vi "Oxford-1820-Main-Launcher.vi"() -> ()   [LabVIEW 2019]
doc: "This VI will launch the PPMS 2 Instrument backend that will contunously monitor the state of the instrument and log to the DSC. The user has the option of launching a user interface (default) or allowing the backend to run headless. Run \"Launch PPMS2 UI.vi\" here or on a different computer to have a remote user interface. You can also use the APIs like \"Get Temperturature\" interact programmatically with the PPMS 2 Instrument backend."
uses:
  <vilib>/JKI/JKI SMO/SMO/Typedefs/SMOState --Enum.ctl
  SMOs/Instrument.Oxford1820/Instrument.Oxford1820.lvclass
  C:/Program Files (x86)/National Instruments/LabVIEW 2019/vi.lib/JKI/JKI SMO/SMO/SMO.lvclass
  C:/Program Files (x86)/National Instruments/LabVIEW 2019/user.lib/LevyLab/Instrument Framework/SMOs/Instrument/Instrument.lvclass
  SMOs/Instrument.Oxford1820 UI/Instrument UI.Oxford1820.lvclass
  C:/Program Files (x86)/National Instruments/LabVIEW 2019/vi.lib/JKI/JKI SMO/SMO.UI/SMO.UI.lvclass
  C:/Program Files (x86)/National Instruments/LabVIEW 2019/user.lib/LevyLab/Instrument Framework/SMOs/Instrument UI/Instrument UI.lvclass
  <vilib>/JKI/JKI SMO/SMO/SMO.lvclass/SMO.ctl
  <vilib>/JKI/JKI SMO/SMO.UI/SMO.UI.lvclass/SMO.UI.ctl
  <vilib>/JKI/JKI SMO/SMO/Private/ReftoDVR--SMO.vi
  <vilib>/JKI/JKI SMO/SMO.UI/SMO.UI.ReftoDVR.vi
  <vilib>/JKI/JKI SMO/SMO/SMO.lvclass
  <vilib>/JKI/JKI SMO/SMO.UI/SMO.UI.lvclass
  <userlib>/LevyLab/Instrument Framework/SMOs/Instrument UI/Instrument UI.lvclass
panel:
  in  "Debug Mode?":bool
  in  "Stop":bool=TRUE
  in  "Start":bool=TRUE
  in  "Splash Status":string="Push Start to Start..." caption="String"
  out "UI SMO State":T1=enum."Stopped"
  out "SMO State":T1
  out "error out":errorcluster
  # "OI 1820"
  # "v"
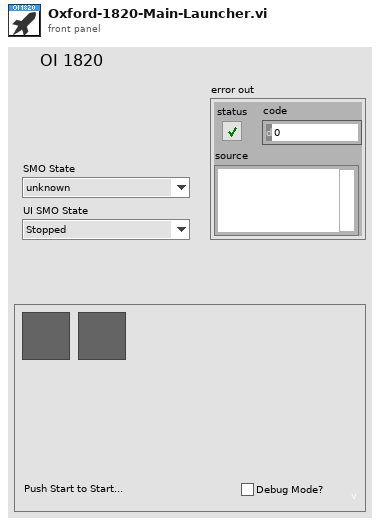
[diagram p1: front panel]
types:
  T1 = typedef "SMO.lvclass/SMOState --Enum.ctl" = enum16{"unknown", "Created", "Started", "Stopped"}
  T2 = enum32{"Invalid", "Standard", "Closed", "Hidden", "Minimized", "Maximized"}
  T3 = enum32{"invalid app kind", "Development System", "Run Time System", "Student Edition", "Embedded LabVIEW", "Evaluation", "Custom"}
  T4 = cluster{"Core":cluster{"Current VI Reference":refnum<vi>, "Close Panel on Exit?":bool}, "Instrument.Oxford1820":refnum<class "Instrument.Oxford1820.lvclass">, "Instrument.Oxford1820 UI":refnum<class "Instrument UI.Oxford1820.lvclass">}
  T5 = cluster{"Current VI Reference":refnum<vi>, "Close Panel on Exit?":bool}
  T6 = typedef "SMO.lvclass/Public Events.ctl" = cluster{"Error":refnum<user-event>, "State":refnum<user-event>, "Reserve State":refnum<user-event>}
  T7 = typedef "SMO.UI.lvclass/PublicEvents--Cluster.ctl" = cluster{"UI Hidden":refnum<user-event>, "UI State":refnum<user-event>}
  T8 = cluster{"Event Registration Refnum":refnum<event-registration>, "Event Registration Refnum":refnum<event-registration>}
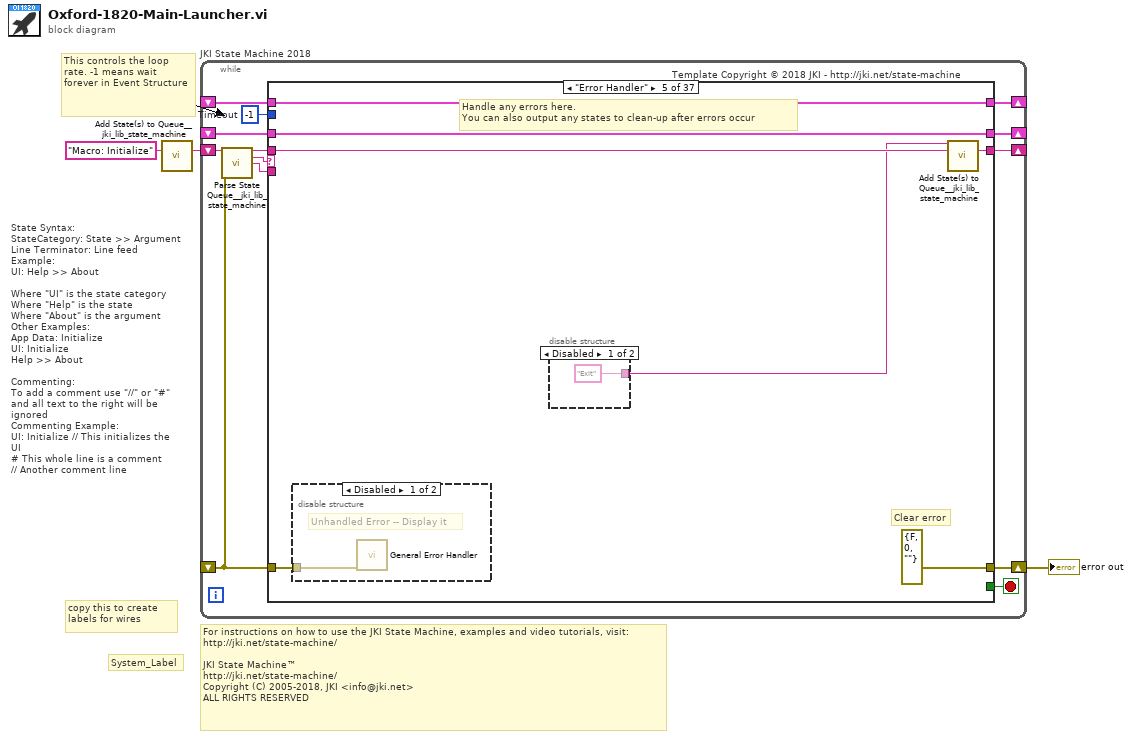
[diagram p0: block diagram]
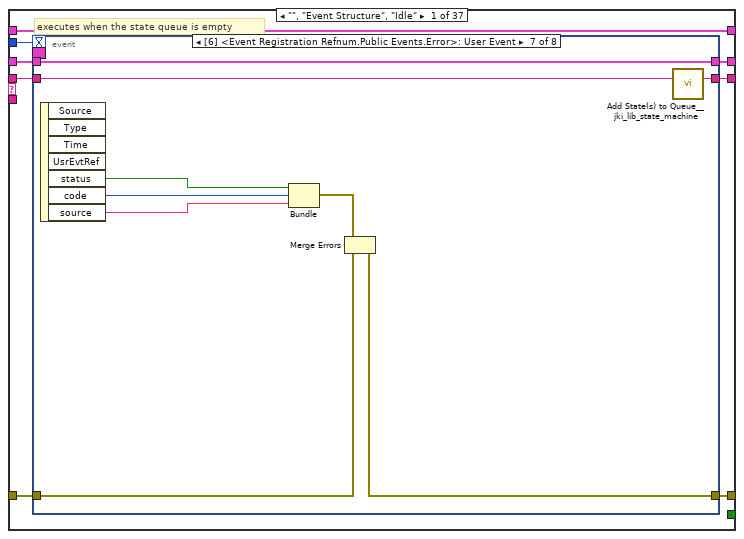
[diagram p2: hidden frame]
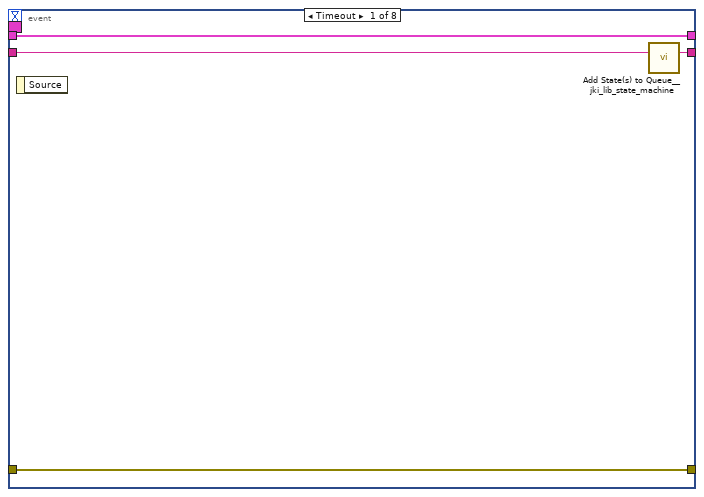
[diagram p3: hidden frame]
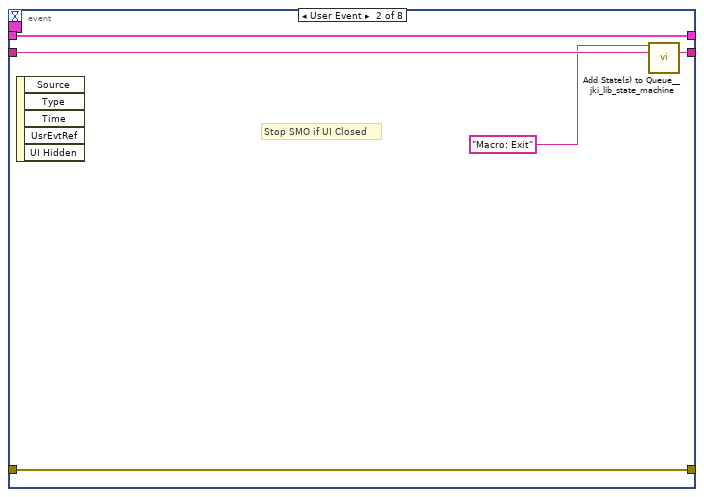
[diagram p4: hidden frame]
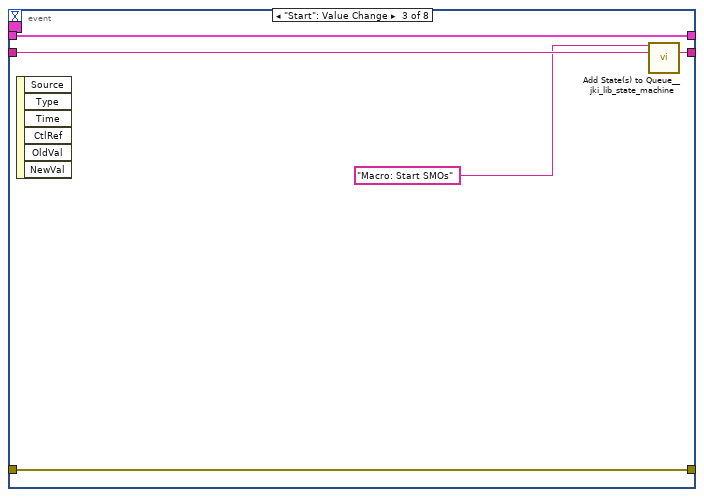
[diagram p5: hidden frame]
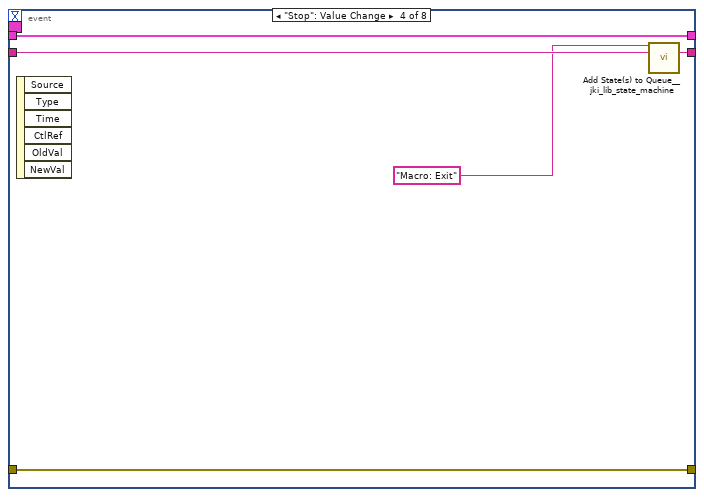
[diagram p6: hidden frame]
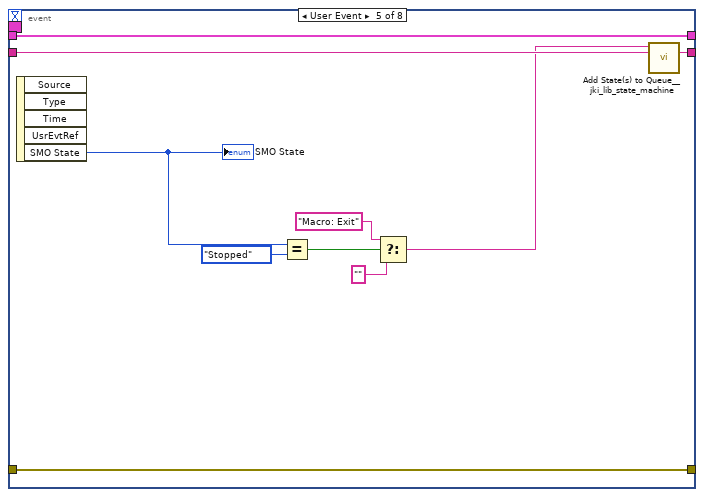
[diagram p7: hidden frame]
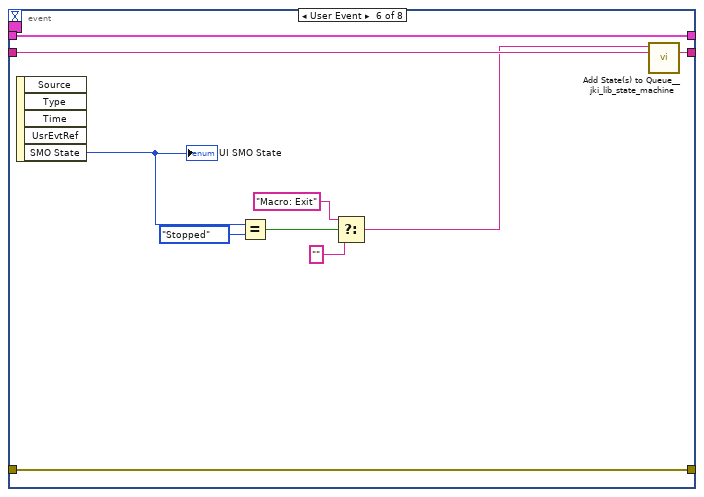
[diagram p8: hidden frame]
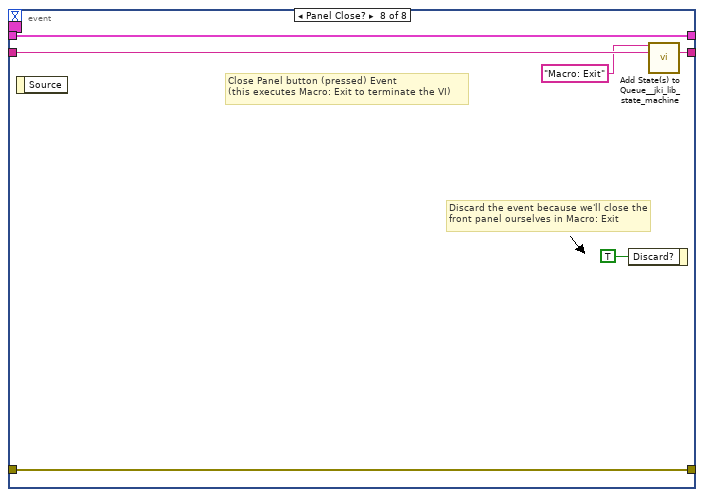
[diagram p9: hidden frame]
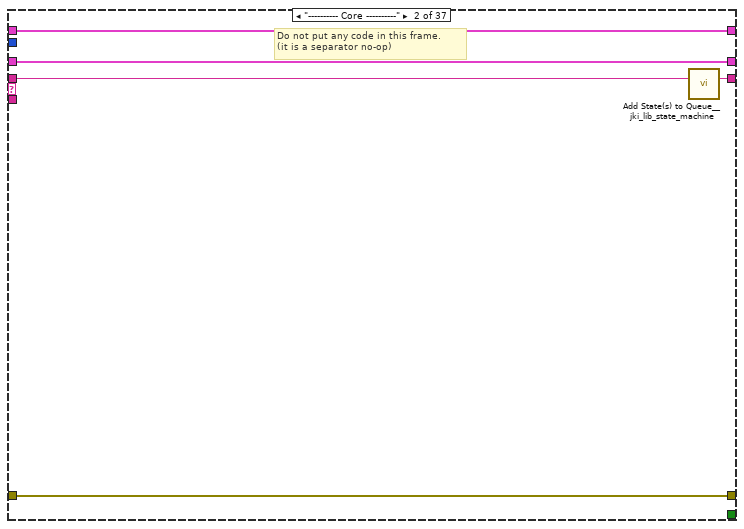
[diagram p10: hidden frame]
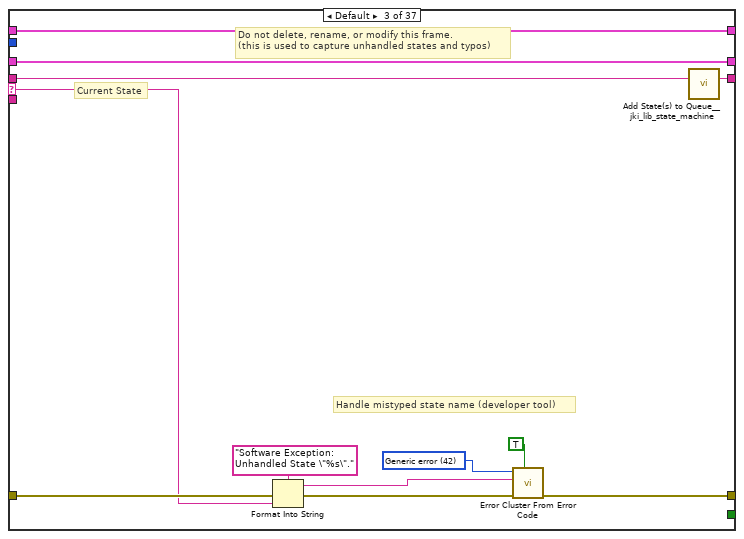
[diagram p11: hidden frame]
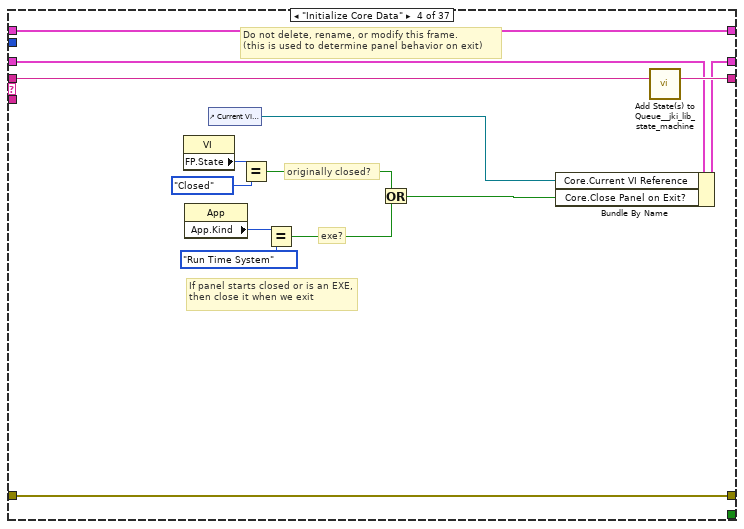
[diagram p12: hidden frame]
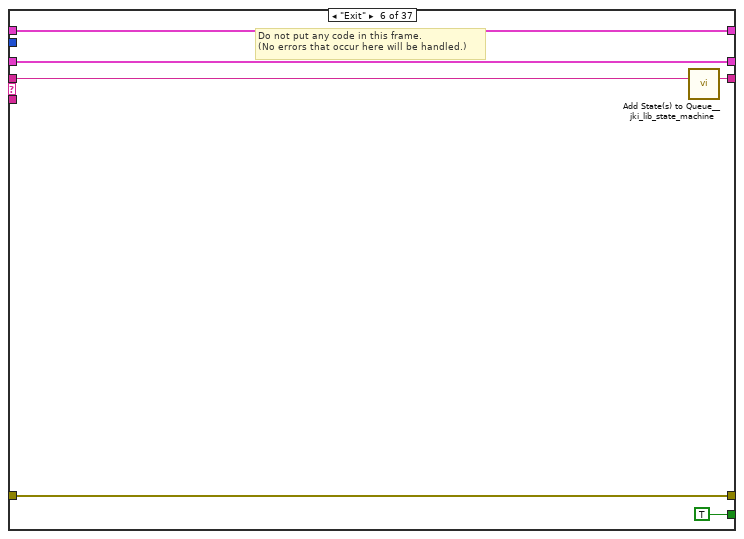
[diagram p15: hidden frame]
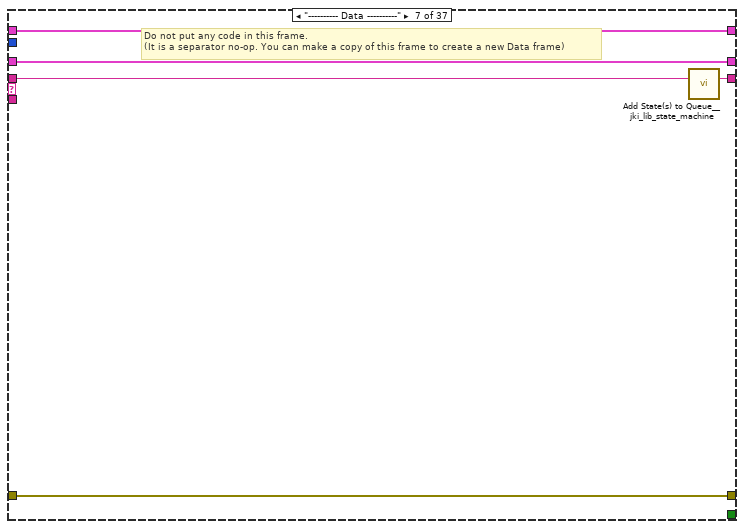
[diagram p16: hidden frame]
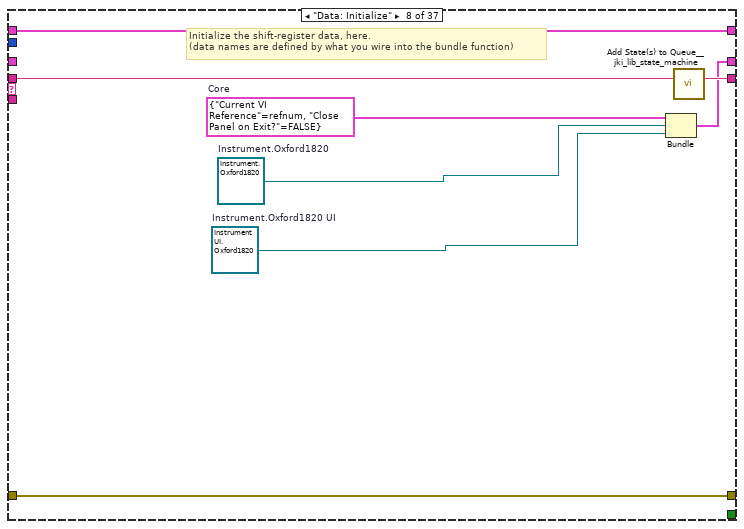
[diagram p17: hidden frame]
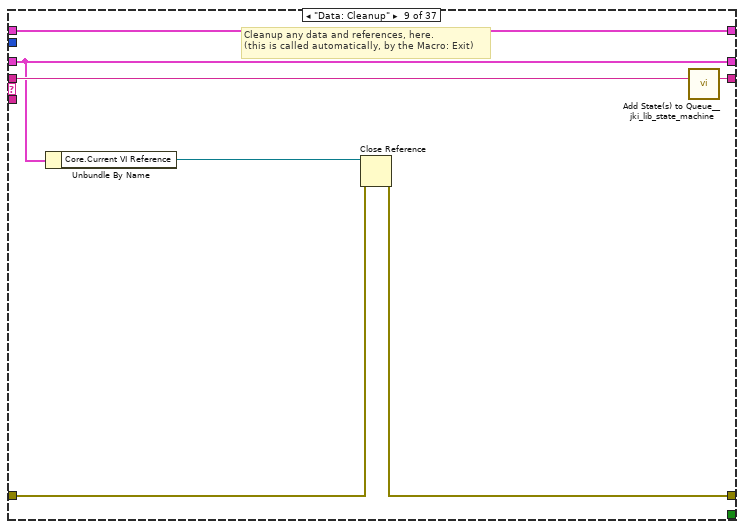
[diagram p18: hidden frame]
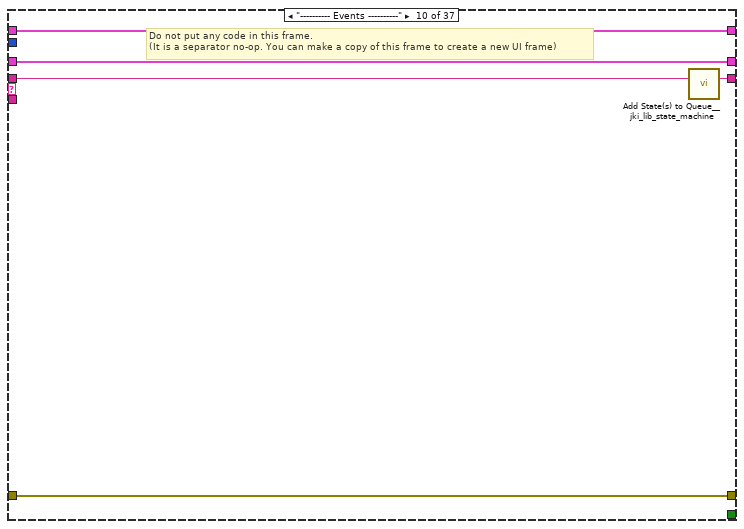
[diagram p19: hidden frame]
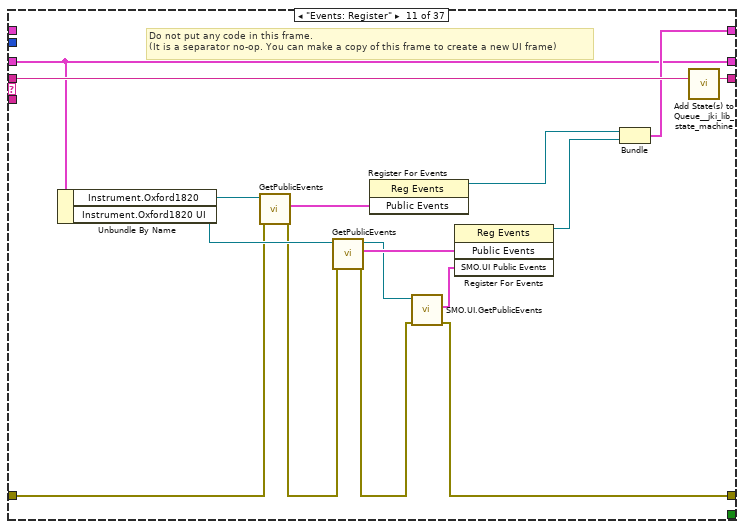
[diagram p20: hidden frame]
diagram:
  # "For instructions on how to use the JKI State Machine, examples and video tutorials, visit:\nhttp://jki.net/state-machine/\n\nJKI State Machine™\nhttp://jki.net/state-machine/\nCopyright (C) 2005-2018, JKI <info@jki.net>\nALL RIGHTS RESERVED"
  # "State Syntax:\nStateCategory: State >> Argument\nLine Terminator: Line feed\nExample:\nUI: Help >> About\n\nWhere \"UI\" is the state category\nWhere \"Help\" is the state\nWhere \"About\" is the argument\nOther Examples:\nApp Data: Initialize\nUI: Initialize\nHelp >> About\n\nCommenting:\nTo add a comment use \"//\" or \"#\" and all text to the right will be ignored\nCommenting Example:\nUI: Initialize // This initializes the UI\n# This whole line is a comment\n// Another comment line"
  # "copy this to create labels for wires"
  # "This controls the loop rate. -1 means wait forever in Event Structure"
  # "System_Label"
  n1 = call <vilib>:"Add State(s) to Queue__jki_lib_state_machine.vi"("State(s) in (\"\")"="Macro: Initialize") -> ("States Out"=w3:string)  [unwired: 14 in]
  n2 = while "JKI State Machine 2018" {
    shift-right: [w9] -> _
    shift-left: _ -> [w4]
    shift-right: [w12] -> w1
    shift-left: _ -> [w7]
    shift-right: [w11] -> _
    shift-left: w3 -> [w13]
    shift-right: [w6] -> _
    shift-left: _ -> [w5]
    stop <- w10 stop-if-true
    w8 = -1  # Timeout
    # "Template Copyright © 2018 JKI - http://jki.net/state-machine"
    n3 = call <vilib>:"Parse State Queue__jki_lib_state_machine.vi"("State Queue"=w13, "Error In (no error)"=w7) -> ("Remaining States"=w15:string, "Current State"=w16:string, "Arguments"=w14:string)  [unwired: 11 in]
    n4 = case shown="\"Error Handler\"" w16 {
      selector: w16 -> [_ _ w85 _ _ _ _ _ _ _ _ _ _ _ _ _ _ _ _ _ _ _ _ _ _ _ _ _ _ _ _ _ _ _ _ _ _]
      tunnel: w15 -> [w24 w83 w89 w109 w116 w124 w129 w137 w144 w149 w165 w171 w176 w182 w189 w201 w279 w284 w289 w295 w301 w307 w319 w324 w335 w344 w355 w370 w384 w391 w402 w417 w432 w447 w456 w463 w468]
      tunnel: w14 -> [_ _ _ _ _ _ _ _ _ _ _ _ _ _ w184 w195 _ _ _ _ _ _ _ _ _ _ _ _ _ _ _ _ _ _ _ w460 _]
      tunnel: [w21 w81 w91 w106 errorcluster {"status"=FALSE, "code"=0, "source"=""} ("error out") w121 w127 w134 w140 w147 w150 w166 w174 w177 w185 w198 w269 w282 w287 w293 w299 w305 w317 w322 w325 w337 w351 w366 w376 w385 w398 w413 w429 w444 w454 w458 w466] -> w12
      tunnel: w7 -> [w20 w81 w90 w106 w112 w121 w127 w134 w141 w147 w156 w167 w174 w179 w186 w199 w270 w282 w287 w293 w299 w305 w317 w322 w329 w338 w347 w362 w377 w386 w395 w410 w427 w440 w454 w459 w466]
      tunnel: [w23 w82 w88 w108 w115 w123 w128 w136 w143 w148 w164 w170 w175 w181 w188 w200 w278 w283 w288 w294 w300 w306 w318 w323 w334 w343 w354 w369 w383 w390 w401 w416 w431 w446 w455 w462 w467] -> w11
      tunnel: [_ _ _ _ _ TRUE _ _ _ _ _ _ _ _ _ _ _ _ _ _ _ _ _ _ _ _ _ _ _ _ _ _ _ _ _ _ _] -> w10
      tunnel: [w19 w80 w87 w107 w113 w122 w126 w135 w139 w146 w159 w169 w173 w180 w187 w197 w267 w281 w286 w292 w298 w304 w316 w321 w332 w339 w352 w367 w380 w388 w399 w414 w428 w443 w453 w461 w465] -> w9
      tunnel: w8 -> [w18 _ _ _ _ _ _ _ _ _ _ _ _ _ _ _ _ _ _ _ _ _ _ _ _ _ _ _ _ _ _ _ _ _ _ _ _]
      tunnel: [w17 w79 w84 w96 w110 w119 w125 w132 w138 w145 w162 w168 w172 w178 w183 w194 w268 w280 w285 w290 w297 w303 w310 w320 w333 w342 w353 w368 w382 w389 w400 w415 w430 w445 w452 w457 w464] -> w6
      tunnel: w5 -> [w17 w79 w84 w96 w110 w119 w125 w132 w138 w145 _ w168 w172 w178 w183 w194 w268 w280 w285 w290 w297 w303 w310 w320 w333 w342 w353 w368 w382 w389 w400 w415 w430 w445 w452 w457 w464]
      tunnel: w4 -> [w22 w80 w87 w102 w113 w122 w126 _ w139 w146 w159 w169 w173 w180 w187 w197 w267 w281 w286 w292 w298 w304 w316 w321 w331 w340 w352 w367 w381 w388 w399 w414 w428 w443 w453 w461 w465]
      frame "", "Event Structure", "Idle" {
        # "executes when the state queue is empty"
        n5 = event shown="[6] <Event Registration Refnum.Public Events.Error>: User Event" {
          selector: w17 -> [_ _ _ _ _ _ _ _]
          dyn-events: _ -> [_ _ _ _ _ _ _ _]
          timeout: w18 -> [_ _ _ _ _ _ _ _]
          tunnel: w24 -> [w28 w33 w38 w43 w53 w63 w72 w78]
          tunnel: [w27 w32 w37 w42 w52 w62 w71 w77] -> w23
          tunnel: w22 -> [w25 w30 w35 w40 w50 w60 w70 w75]
          tunnel: [w26 w31 w36 w41 w51 w61 w65 w76] -> w21
          tunnel: w20 -> [w26 w31 w36 w41 w51 w61 w66 w76]
          tunnel: [w25 w30 w35 w40 w50 w60 w70 w75] -> w19
          event Timeout {
            n6 = event-data() -> ()  [unwired: 1 in, 1 out]
            n7 = call <vilib>:"Add State(s) to Queue__jki_lib_state_machine.vi"("State(s) in (\"\")"=w28) -> ("States Out"=w27:string)  [unwired: 14 in]
          }
          event User Event {
            # "Stop SMO if UI Closed"
            n8 = event-data() -> ()  [unwired: 1 in, 5 out]
            n9 = call <vilib>:"Add State(s) to Queue__jki_lib_state_machine.vi"("State(s) in Front (\"\")"="Macro: Exit" ("State(s) in Front (\"\")"), "State(s) in (\"\")"=w33) -> ("States Out"=w32:string)  [unwired: 13 in]
          }
          event "Start": Value Change {
            n10 = event-data() -> ()  [unwired: 1 in, 6 out]
            n11 = call <vilib>:"Add State(s) to Queue__jki_lib_state_machine.vi"("State(s) in Front (\"\")"="Macro: Start SMOs" ("State(s) in Front (\"\")"), "State(s) in (\"\")"=w38) -> ("States Out"=w37:string)  [unwired: 13 in]
          }
          event "Stop": Value Change {
            n12 = event-data() -> ()  [unwired: 1 in, 6 out]
            n13 = call <vilib>:"Add State(s) to Queue__jki_lib_state_machine.vi"("State(s) in Front (\"\")"="Macro: Exit" ("State(s) in Front (\"\")"), "State(s) in (\"\")"=w43) -> ("States Out"=w42:string)  [unwired: 13 in]
          }
          event User Event {
            n14 = event-data() -> ("SMO State"=w45:T1)  [unwired: 1 in, 4 out]
            "SMO State" <- w45
            n15 = Equal?(x=w45, y=SMOState_--Enum."Stopped") -> (x = y?=w48:bool)
            n16 = Select(t="Macro: Exit", s=w48, f="" ("State(s) in Front (\"\")")) -> (s? t:f=w44:string)
            n17 = call <vilib>:"Add State(s) to Queue__jki_lib_state_machine.vi"("State(s) in Front (\"\")"=w44, "State(s) in (\"\")"=w53) -> ("States Out"=w52:string)  [unwired: 13 in]
          }
          event User Event {
            n18 = event-data() -> ("SMO State"=w54:T1)  [unwired: 1 in, 4 out]
            "UI SMO State" <- w54
            n19 = Equal?(x=w54, y=SMOState_--Enum."Stopped") -> (x = y?=w58:bool)
            n20 = Select(t="Macro: Exit", s=w58, f="" ("State(s) in Front (\"\")")) -> (s? t:f=w56:string)
            n21 = call <vilib>:"Add State(s) to Queue__jki_lib_state_machine.vi"("State(s) in Front (\"\")"=w56, "State(s) in (\"\")"=w63) -> ("States Out"=w62:string)  [unwired: 13 in]
          }
          event User Event {
            n22 = event-data() -> ("status"=w67:bool, "code"=w69:i32, "source"=w68:string)  [unwired: 1 in, 4 out]
            n23 = Bundle("status"=w67, "code"=w69, "source"=w68) -> (w64:errorcluster)  [unwired: 1 in]
            n24 = Merge Errors(w64, w66) -> (w65:errorcluster)
            n25 = call <vilib>:"Add State(s) to Queue__jki_lib_state_machine.vi"("State(s) in (\"\")"=w72) -> ("States Out"=w71:string)  [unwired: 14 in]
          }
          event Panel Close? {
            # "Discard the event because we'll close the front panel ourselves in Macro: Exit"
            # "Close Panel button (pressed) Event\n(this executes Macro: Exit to terminate the VI)"
            n26 = event-data() -> ()  [unwired: 1 in, 1 out]
            n27 = event-data("Discard?"=TRUE) -> ()  [unwired: 1 in, 1 out]
            n28 = call <vilib>:"Add State(s) to Queue__jki_lib_state_machine.vi"("State(s) in Front (\"\")"="Macro: Exit", "State(s) in (\"\")"=w78) -> ("States Out"=w77:string)  [unwired: 13 in]
          }
        }
      }
      frame "---------- Core ----------" {
        # "Do not put any code in this frame.\n(it is a separator no-op)"
        n29 = call <vilib>:"Add State(s) to Queue__jki_lib_state_machine.vi"("State(s) in (\"\")"=w83) -> ("States Out"=w82:string)  [unwired: 14 in]
      }
      frame Default {
        w94 = 42 items=["No error", "Argument error", "Memory is full", "Out of zone", "End of file", "File already open", "Generic file I/O error", "File not found", "File permission error", "Disk is full", "Duplicate path", "Too many files open", "System feature not enabled", "Resource file not found", "Cannot add resource", "Resource not found", "Image not found", "Image memory error", "Pen does not exist", "Config type invalid", "Config token not found", "Config parse error", "Config memory error", "Bad external code format", "Bad external code offset", "External code not present", "Null window", "Destroy window error", "Null menu", "Print aborted", "Bad print record", "Print driver error", "Windows error during printing", "Memory error during printing", "Print dialog error", "Generic print error", "Invalid device refnum", "Device not found", "Device parameter error", "Device unit error", "Cannot open device", "Device call aborted", "Generic error", "Cancelled by user", "Object ID too low", "Object ID too high", "Object not in heap", "Unknown heap", "Unknown object (invalid DefProc)", "Unknown object (DefProc not in table)", "Message out of range", "Invalid (null) method", "Unknown message", "Manager call not supported", "Bad address", "Network operation in progress", "Network operation timed out", "Connection is busy", "Network attribute not supported", "Network error", "Address in use", "System out of memory", "Connection aborted", "Connection refused", "Not connected", "Already connected", "Connection closed", "Initialization error (interapplication manager)", "Bad occurrence", "Wait on unbound occurrence handler", "Occurrence queue overflow", "Datalog type conflict", "Unused", "Unrecognized type (interapplication manager)", "Memory corrupt", "Failed to make temporary DLL", "Old CIN version", "Drag socket not found", "Failed to load drop-object", "Failed to register OLE object", "Failed to release OLE object", "Format specifier type mismatch", "Unknown format specifier", "Too few format specifiers", "Too many format specifiers", "Scan failed", "Newer CIN version", "Error converting to variant", "Runtime menu error", "Password tampered", "Variant attribute not found", "Incompatible variant data type", "Event data is not available", "Event Store is not present", "Occurrence is not found", "Event Queue is not created", "Event info is not available", "Refnum passed is NULL", "Error retrieving Class GUID", "Error retrieving CoClass GUID", "Error retrieving TypeLib GUID.", "Bad built application magic bytes.", "Specific driver is different from the specific driver associated with the Logical Name.", "There is no session opened to the class driver.", "Max Error", "MAX - Error with config objects", "MAX - Error loading configuration", "MAX - Group not supported"]
        # "Current State"
        # "Do not delete, rename, or modify this frame.\n(this is used to capture unhandled states and typos)"
        # "Handle mistyped state name (developer tool)"
        n30 = Format Into String(format string="Software Exception: Unhandled State \"%s\"." ("message"), error in=w90, w85) -> (resulting string=w93:string, error out=w92:errorcluster)  [unwired: 1 in]
        n31 = call <vilib>:"Error Cluster From Error Code.vi"("show call chain? (False)"=TRUE, "error in (no error)"=w92, "error message (\"\")"=w93, "error code (0)"=w94) -> ("error out"=w91:errorcluster)  [unwired: 5 in]
        n32 = call <vilib>:"Add State(s) to Queue__jki_lib_state_machine.vi"("State(s) in (\"\")"=w89) -> ("States Out"=w88:string)  [unwired: 14 in]
      }
      frame "Initialize Core Data" {
        # "Do not delete, rename, or modify this frame.\n(this is used to determine panel behavior on exit)"
        # "originally closed?"
        # "exe?"
        # "If panel starts closed or is an EXE, then close it when we exit"
        n33 = property class="VI"() -> ("FP.State"=w99:T2)  [unwired: 2 in, 2 out]
        n34 = property class="App"() -> ("App.Kind"=w105:T3)  [unwired: 2 in, 2 out]
        n35 = control-ref of="Current VI Reference"() -> (w100:refnum<vi>)
        n36 = Equal?(x=w99, y=T2."Closed" ("Front Panel Window:State")) -> (x = y?=w97:bool)
        n37 = Equal?(x=w105, y=T3."Run Time System" ("Application:Kind")) -> (x = y?=w103:bool)
        n38 = Or(x=w97, y=w103) -> (x .or. y?=w101:bool)
        n39 = Bundle By Name(cluster=w102, "Core.Current VI Reference"=w100, "Core.Close Panel on Exit?"=w101) -> (w107:T4)
        n40 = call <vilib>:"Add State(s) to Queue__jki_lib_state_machine.vi"("State(s) in (\"\")"=w109) -> ("States Out"=w108:string)  [unwired: 14 in]
      }
      frame "Error Handler" {
        # "Handle any errors here.\nYou can also output any states to clean-up after errors occur"
        # "Clear error"
        n41 = disable-structure shown="Disabled" {
          disable-tunnel: w112 -> [w118 _]
          frame Disabled {
            # "Unhandled Error -- Display it"
            n42 = call <vilib>:"General Error Handler.vi"("error in (no error)"=w118) -> ()  [unwired: 10 in, 5 out]
          }
          frame Enabled {
          }
        }
        n43 = disable-structure shown="Disabled" {
          disable-tunnel: ["Exit" _] -> w111
          frame Disabled {
          }
          frame Enabled {
          }
        }
        n44 = call <vilib>:"Add State(s) to Queue__jki_lib_state_machine.vi"("State(s) in Front (\"\")"=w111, "State(s) in (\"\")"=w116) -> ("States Out"=w115:string)  [unwired: 13 in]
      }
      frame "Exit" {
        # "Do not put any code in this frame.\n(No errors that occur here will be handled.)"
        n45 = call <vilib>:"Add State(s) to Queue__jki_lib_state_machine.vi"("State(s) in (\"\")"=w124) -> ("States Out"=w123:string)  [unwired: 14 in]
      }
      frame "---------- Data ----------" {
        # "Do not put any code in this frame.\n(It is a separator no-op. You can make a copy of this frame to create a new Data frame)"
        n46 = call <vilib>:"Add State(s) to Queue__jki_lib_state_machine.vi"("State(s) in (\"\")"=w129) -> ("States Out"=w128:string)  [unwired: 14 in]
      }
      frame "Data: Initialize" {
        w131 = refnum<class "Instrument UI.Oxford1820.lvclass"> refnum  # Instrument.Oxford1820 UI
        w130 = refnum<class "Instrument.Oxford1820.lvclass"> refnum  # Instrument.Oxford1820
        w133 = T5 {"Current VI Reference"=refnum, "Close Panel on Exit?"=FALSE}  # Core
        # "Initialize the shift-register data, here.\n(data names are defined by what you wire into the bundle function)"
        n47 = Bundle("Core"=w133, "Instrument.Oxford1820"=w130, "Instrument.Oxford1820 UI"=w131) -> (w135:T4)  [unwired: 1 in]
        n48 = call <vilib>:"Add State(s) to Queue__jki_lib_state_machine.vi"("State(s) in (\"\")"=w137) -> ("States Out"=w136:string)  [unwired: 14 in]
      }
      frame "Data: Cleanup" {
        # "Cleanup any data and references, here.\n(this is called automatically, by the Macro: Exit)"
        n49 = Unbundle By Name(w139) -> ("Core.Current VI Reference"=w142:refnum<vi>)
        n50 = Close Reference(reference=w142, error in (no error)=w141) -> (error out=w140:errorcluster)
        n51 = call <vilib>:"Add State(s) to Queue__jki_lib_state_machine.vi"("State(s) in (\"\")"=w144) -> ("States Out"=w143:string)  [unwired: 14 in]
      }
      frame "---------- Events ----------" {
        # "Do not put any code in this frame.\n(It is a separator no-op. You can make a copy of this frame to create a new UI frame)"
        n52 = call <vilib>:"Add State(s) to Queue__jki_lib_state_machine.vi"("State(s) in (\"\")"=w149) -> ("States Out"=w148:string)  [unwired: 14 in]
      }
      frame "Events: Register" {
        # "Do not put any code in this frame.\n(It is a separator no-op. You can make a copy of this frame to create a new UI frame)"
        n53 = Unbundle By Name(w159) -> ("Instrument.Oxford1820"=w158:refnum<class "Instrument.Oxford1820.lvclass">, "Instrument.Oxford1820 UI"=w157:refnum<class "Instrument UI.Oxford1820.lvclass">)
        n54 = call <vilib>:"GetPublicEvents.vi"("error in (no error)"=w156, "SMO"=w158) -> ("error out"=w155:errorcluster, "Public Events"=w160:T6)  [unwired: 7 in, 1 out]
        n55 = call <vilib>:"GetPublicEvents.vi"("error in (no error)"=w155, "SMO"=w157) -> ("error out"=w151:errorcluster, "Public Events"=w161:T6, "SMO out"=w153:refnum<class "Instrument UI.Oxford1820.lvclass">)  [unwired: 7 in]
        n56 = register-events(w160) -> (reference out=w163:refnum<event-registration>)  [unwired: 2 in, 1 out]
        n57 = call <vilib>:"SMO.UI.GetPublicEvents.vi"("error in (no error)"=w151, "SMO.UI"=w153) -> ("error out"=w150:errorcluster, "SMO.UI Public Events"=w152:T7)  [unwired: 7 in, 1 out]
        n58 = register-events(w161, w152) -> (reference out=w154:refnum<event-registration>)  [unwired: 2 in, 1 out]
        n59 = Bundle("Event Registration Refnum"=w163, "Event Registration Refnum"=w154) -> (w162:T8)  [unwired: 1 in]
        n60 = call <vilib>:"Add State(s) to Queue__jki_lib_state_machine.vi"("State(s) in (\"\")"=w165) -> ("States Out"=w164:string)  [unwired: 14 in]
      }
      frame "Events: Unregister" {
        # "Do not put any code in this frame.\n(It is a separator no-op. You can make a copy of this frame to create a new UI frame)"
        n61 = Unregister For Events(event registration refnum=w168, error in=w167) -> (error out=w166:errorcluster)
        n62 = call <vilib>:"Add State(s) to Queue__jki_lib_state_machine.vi"("State(s) in (\"\")"=w171) -> ("States Out"=w170:string)  [unwired: 14 in]
      }
      frame "---------- UI ----------" {
        # "Do not put any code in this frame.\n(It is a separator no-op. You can make a copy of this frame to create a new UI frame)"
        n63 = call <vilib>:"Add State(s) to Queue__jki_lib_state_machine.vi"("State(s) in (\"\")"=w176) -> ("States Out"=w175:string)  [unwired: 14 in]
      }
      frame "UI: Initialize" {
        # "Initialize the User Interface, here.\n(this is called automatically, by the Macro: Init)"
        n64 = invoke on="Stop" class="Bool (strict)" method="Reinit To Default"() -> ()  [unwired: 3 in, 3 out]
        n65 = invoke on="error out" class="Clust (strict)" method="Reinit To Default"() -> ()  [unwired: 3 in, 3 out]
        n66 = invoke on="SMO State" class="Enum (strict)" method="Reinit To Default"() -> ()  [unwired: 3 in, 3 out]
        n67 = invoke on="Start" class="Bool (strict)" method="Reinit To Default"() -> ()  [unwired: 3 in, 3 out]
        n68 = call <userlib>:"Fit VI window to Largest Dec__ogtk.vi"("error in (no error)"=w179) -> ("error out"=w177:errorcluster)  [unwired: 5 in, 1 out]
        n69 = call <vilib>:"Add State(s) to Queue__jki_lib_state_machine.vi"("State(s) in (\"\")"=w182) -> ("States Out"=w181:string)  [unwired: 14 in]
      }
      frame "UI: Cursor Set" {
        # "Argument"
        # "Set and Unset Cursor Busy.\n(Usage: \"UI: Cursor Set >> Busy|Idle\")"
        n70 = case shown="\"Idle\", Default" w184 {
          tunnel: w186 -> [w191 w193]
          tunnel: [w190 w192] -> w185
          frame "Idle", Default {
            n71 = call <vilib>:"Unset Busy.vi"("error in (no error)"=w191) -> ("error out"=w190:errorcluster)  [unwired: 10 in]
          }
          frame "Busy" {
            n72 = call <vilib>:"Set Busy.vi"("error in (no error)"=w193) -> ("error out"=w192:errorcluster)  [unwired: 9 in, 1 out]
          }
        }
        n73 = call <vilib>:"Add State(s) to Queue__jki_lib_state_machine.vi"("State(s) in (\"\")"=w189) -> ("States Out"=w188:string)  [unwired: 14 in]
      }
      frame "UI: Front Panel State" {
        # "Argument"
        # "Set Front Panel Open or Closed\n(Usage: \"UI: Front Panel State >> Open|Close\")"
        n74 = Unbundle By Name(w197) -> ("Core.Current VI Reference"=w196:refnum<vi>)
        n75 = case shown="\"Open\", \"Standard\", Default" w195 {
          tunnel: w199 -> [w207 w222 w233 w246 w259]
          tunnel: [w209 w223 w235 w248 w261] -> w198
          tunnel: w196 -> [w208 w220 w234 w247 w260]
          frame "Open", "Standard", Default {
            w202 = T2."Standard" ("State")
            n76 = property class="VI"(reference=w208, error in=w207) -> (reference out=w205:refnum<vi>, error out=w206:errorcluster, "FP.State"=w204:T2)
            n77 = Not Equal?(x=w204, y=w202) -> (x != y?=w203:bool)
            n78 = case shown="False" w203 {
              tunnel: [w213 w215] -> w209
              tunnel: w206 -> [w212 w215]
              tunnel: w205 -> [w211 _]
              tunnel: w202 -> [w210 _]
              frame True {
                n79 = invoke class="VI" method="FP.Open"(reference=w211, error in=w212, "Activate"=TRUE, "State"=w210) -> (error out=w213:errorcluster)  [unwired: 1 in, 4 out]
              }
              frame False {
              }
            }
          }
          frame "Close", "Closed" {
            n80 = property class="VI"(reference=w220, error in=w222) -> (reference out=w219:refnum<vi>, error out=w221:errorcluster, "FP.State"=w217:T2)
            n81 = Not Equal?(x=w217, y=T2."Closed" ("Front Panel Window:State")) -> (x != y?=w216:bool)
            n82 = case shown="True" w216 {
              tunnel: [w224 w227] -> w223
              tunnel: w221 -> [w224 w226]
              tunnel: w219 -> [_ w225]
              frame False {
              }
              frame True {
                n83 = invoke class="VI" method="FP.Close"(reference=w225, error in=w226) -> (error out=w227:errorcluster)  [unwired: 1 in, 2 out]
              }
            }
          }
          frame "Hidden", "Hide" {
            w228 = T2."Hidden" ("State")
            n84 = property class="VI"(reference=w234, error in=w233) -> (reference out=w231:refnum<vi>, error out=w232:errorcluster, "FP.State"=w230:T2)
            n85 = Not Equal?(x=w230, y=w228) -> (x != y?=w229:bool)
            n86 = case shown="True" w229 {
              tunnel: [w239 w240] -> w235
              tunnel: w232 -> [w238 w240]
              tunnel: w231 -> [w237 _]
              tunnel: w228 -> [w236 _]
              frame True {
                n87 = invoke class="VI" method="FP.Open"(reference=w237, error in=w238, "State"=w236) -> (error out=w239:errorcluster)  [unwired: 2 in, 4 out]
              }
              frame False {
              }
            }
          }
          frame "Minimize", "Minimized" {
            w241 = T2."Minimized" ("State")
            n88 = property class="VI"(reference=w247, error in=w246) -> (reference out=w244:refnum<vi>, error out=w245:errorcluster, "FP.State"=w243:T2)
            n89 = Not Equal?(x=w243, y=w241) -> (x != y?=w242:bool)
            n90 = case shown="True" w242 {
              tunnel: [w252 w253] -> w248
              tunnel: w245 -> [w251 w253]
              tunnel: w244 -> [w250 _]
              tunnel: w241 -> [w249 _]
              frame True {
                n91 = invoke class="VI" method="FP.Open"(reference=w250, error in=w251, "State"=w249) -> (error out=w252:errorcluster)  [unwired: 2 in, 4 out]
              }
              frame False {
              }
            }
          }
          frame "Maximize", "Maximized" {
            w254 = T2."Maximized" ("State")
            n92 = property class="VI"(reference=w260, error in=w259) -> (reference out=w257:refnum<vi>, error out=w258:errorcluster, "FP.State"=w256:T2)
            n93 = Not Equal?(x=w256, y=w254) -> (x != y?=w255:bool)
            n94 = case shown="True" w255 {
              tunnel: [w265 w266] -> w261
              tunnel: w258 -> [w264 w266]
              tunnel: w257 -> [w263 _]
              tunnel: w254 -> [w262 _]
              frame True {
                n95 = invoke class="VI" method="FP.Open"(reference=w263, error in=w264, "State"=w262) -> (error out=w265:errorcluster)  [unwired: 2 in, 4 out]
              }
              frame False {
              }
            }
          }
        }
        n96 = call <vilib>:"Add State(s) to Queue__jki_lib_state_machine.vi"("State(s) in (\"\")"=w201) -> ("States Out"=w200:string)  [unwired: 14 in]
      }
      frame "UI: Set Background Color" {
        # "Do not put any code in this frame.\n(It is a separator no-op. You can make a copy of this frame to create a new UI frame)"
        n97 = property class="VI"(error in=w270) -> (error out=w272:errorcluster, "Panel"=w273:refnum<vi>)  [unwired: 1 in, 1 out]
        n98 = property class="Pnl"(reference=w273, error in=w272) -> (error out=w271:errorcluster, "Panes[]"=w274:refnum<vi>[])  [unwired: 1 out]
        n99 = Index Array(array=w274, index=0) -> (element=w276:refnum<vi>)
        n100 = property class="Pane"(reference=w276, error in=w271, "PaneColor"=u32 16777238 ("Color Box")) -> (error out=w269:errorcluster)  [unwired: 1 out]
        n101 = call <vilib>:"Add State(s) to Queue__jki_lib_state_machine.vi"("State(s) in (\"\")"=w279) -> ("States Out"=w278:string)  [unwired: 14 in]
      }
      frame "UI: Exit" {
        # "Do not put any code in this frame.\n(It is a separator no-op. You can make a copy of this frame to create a new UI frame)"
        n102 = invoke on="Start" class="Bool (strict)" method="Reinit To Default"() -> ()  [unwired: 3 in, 3 out]
        n103 = invoke on="Stop" class="Bool (strict)" method="Reinit To Default"() -> ()  [unwired: 3 in, 3 out]
        n104 = call <vilib>:"Add State(s) to Queue__jki_lib_state_machine.vi"("State(s) in (\"\")"=w284) -> ("States Out"=w283:string)  [unwired: 14 in]
      }
      frame "---------- Macro ----------" {
        # "Do not put any code in this frame.\n(It is a separator no-op. You can make a copy of this frame to create a new Macro frame)"
        n105 = call <vilib>:"Add State(s) to Queue__jki_lib_state_machine.vi"("State(s) in (\"\")"=w289) -> ("States Out"=w288:string)  [unwired: 14 in]
      }
      frame "Macro: Initialize" {
        # "Initialization Macro\n(This is called once, when the VI starts)"
        n106 = call <vilib>:"Add State(s) to Queue__jki_lib_state_machine.vi"("State(s) in Front (\"\")"="Data: Initialize\nInitialize Core Data\n//Events: Register\nUI: Initialize\nUI: Front Panel State >> Open\nUI: Set Background Color\nSplash: Set Status >> Push Start to Start...", "State(s) in (\"\")"=w295) -> ("States Out"=w294:string)  [unwired: 13 in]
      }
      frame "Macro: Start SMOs" {
        # "Do not put any code in this frame.\n(It is a separator no-op. You can make a copy of this frame to create a new Macro frame)"
        n107 = call <vilib>:"Add State(s) to Queue__jki_lib_state_machine.vi"("State(s) in Front (\"\")"="Splash: Set Status >> Starting Instrument...\nSMO: Create Instrument\nSMO: Create Instrument UI\nEvents: Register\nSMO: Start Instrument\nSplash: Set Status >> Instrument Process Started...\nSplash: Set Status >> Starting User Interface...\nSMO: Start Instrument UI\nUI: Front Panel State >> Hide\nSMO: Show Instrument UI" ("State(s) in Front (\"\")"), "State(s) in (\"\")"=w301) -> ("States Out"=w300:string)  [unwired: 13 in]
      }
      frame "Macro: Stop SMOs" {
        # "Do not put any code in this frame.\n(It is a separator no-op. You can make a copy of this frame to create a new Macro frame)"
        n108 = call <vilib>:"Add State(s) to Queue__jki_lib_state_machine.vi"("State(s) in Front (\"\")"="SMO: Stop Instrument\nSMO: Destroy Instrument\nSMO: Hide Instrument UI\nSMO: Stop Instrument UI\nSMO: Destroy Instrument UI" ("State(s) in Front (\"\")"), "State(s) in (\"\")"=w307) -> ("States Out"=w306:string)  [unwired: 13 in]
      }
      frame "Macro: Exit" {
        # "Exit Macro\n(This is called once, when the VI exits)"
        n109 = Unbundle By Name(w316) -> ("Core.Close Panel on Exit?"=w315:bool)
        n110 = Select(t="UI: Front Panel State >> Open", s=w315, f="") -> (s? t:f=w312:string)
        n111 = call <vilib>:"Add State(s) to Queue__jki_lib_state_machine.vi"("State(s) in Front (\"\")"="UI: Front Panel State >> Open\nUI: Exit", "State(s) in (\"\")"=w312, "State(s) at Back (\"\")"="Macro: Stop SMOs\nData: Cleanup\nEvents: Unregister\nExit") -> ("States Out"=w311:string)  [unwired: 12 in]
        n112 = call <vilib>:"Add State(s) to Queue__jki_lib_state_machine.vi"("State(s) in Front (\"\")"=w311, "State(s) in (\"\")"=w319) -> ("States Out"=w318:string)  [unwired: 13 in]
      }
      frame "---------- SMO ----------" {
        # "Do not put any code in this frame.\n(It is a separator no-op. You can make a copy of this frame to create a new Macro frame)"
        n113 = call <vilib>:"Add State(s) to Queue__jki_lib_state_machine.vi"("State(s) in (\"\")"=w324) -> ("States Out"=w323:string)  [unwired: 14 in]
      }
      frame "SMO: Create Instrument" {
        # "Do not put any code in this frame.\n(It is a separator no-op. You can make a copy of this frame to create a new Macro frame)"
        n114 = Unbundle By Name(w331) -> ("Instrument.Oxford1820"=w330:refnum<class "Instrument.Oxford1820.lvclass">)
        n115 = call-dynamic "Create Instrument SMO.vi"("error in (no error)"=w329, "Debug Mode? [F]"="Debug Mode?", "Configuration Window? [T]"=FALSE, "Instrument in"=w330) -> ("error out"=w325:errorcluster, "Instrument out"=w326:refnum<class "Instrument.Oxford1820.lvclass">)  [unwired: 6 in]
        n116 = Bundle By Name(cluster=w331, "Instrument.Oxford1820"=w326) -> (w332:T4)
        n117 = call <vilib>:"Add State(s) to Queue__jki_lib_state_machine.vi"("State(s) in (\"\")"=w335) -> ("States Out"=w334:string)  [unwired: 14 in]
      }
      frame "SMO: Start Instrument" {
        # "Do not put any code in this frame.\n(It is a separator no-op. You can make a copy of this frame to create a new Macro frame)"
        n118 = Unbundle By Name(w340) -> ("Instrument.Oxford1820"=w341:refnum<class "Instrument.Oxford1820.lvclass">)
        n119 = call <vilib>:"Start.vi"("error in (no error)"=w338, "SMO"=w341) -> ("error out"=w337:errorcluster, "SMO out"=w336:refnum<class "Instrument.Oxford1820.lvclass">)  [unwired: 8 in]
        n120 = Bundle By Name(cluster=w340, "Instrument.Oxford1820"=w336) -> (w339:T4)
        n121 = call <vilib>:"Add State(s) to Queue__jki_lib_state_machine.vi"("State(s) in (\"\")"=w344) -> ("States Out"=w343:string)  [unwired: 14 in]
      }
      frame "SMO: Stop Instrument" {
        # "Do not put any code in this frame.\n(It is a separator no-op. You can make a copy of this frame to create a new Macro frame)"
        n122 = Unbundle By Name(w352) -> ("Instrument.Oxford1820"=w350:refnum<class "Instrument.Oxford1820.lvclass">)
        n123 = call <vilib>:"GetState.vi"("error in (no error)"=w347, "SMO"=w350) -> ("error out"=w346:errorcluster, "SMO State"=w349:T1, "SMO out"=w345:refnum<class "Instrument.Oxford1820.lvclass">)  [unwired: 7 in]
        n124 = call <vilib>:"Clear Errors.vi"("error in (no error)"=w346) -> ("error out"=w348:errorcluster)  [unwired: 5 in, 1 out]
        n125 = case shown="\"Created\", \"Started\"" w349 {
          tunnel: [w356 w359] -> w351
          tunnel: w348 -> [w356 w358]
          tunnel: w345 -> [_ w357]
          frame Default {
          }
          frame "Created", "Started" {
            n126 = call <vilib>:"Stop.vi"("error in (no error)"=w358, "SMO"=w357) -> ("error out"=w359:errorcluster)  [unwired: 8 in, 1 out]
          }
        }
        n127 = call <vilib>:"Add State(s) to Queue__jki_lib_state_machine.vi"("State(s) in (\"\")"=w355) -> ("States Out"=w354:string)  [unwired: 14 in]
      }
      frame "SMO: Destroy Instrument" {
        # "Do not put any code in this frame.\n(It is a separator no-op. You can make a copy of this frame to create a new Macro frame)"
        n128 = Unbundle By Name(w367) -> ("Instrument.Oxford1820"=w365:refnum<class "Instrument.Oxford1820.lvclass">)
        n129 = call <vilib>:"GetState.vi"("error in (no error)"=w362, "SMO"=w365) -> ("error out"=w361:errorcluster, "SMO State"=w364:T1, "SMO out"=w360:refnum<class "Instrument.Oxford1820.lvclass">)  [unwired: 7 in]
        n130 = call <vilib>:"Clear Errors.vi"("error in (no error)"=w361) -> ("error out"=w363:errorcluster)  [unwired: 5 in, 1 out]
        n131 = case shown="\"Stopped\"" w364 {
          tunnel: [w371 w374] -> w366
          tunnel: w363 -> [w371 w373]
          tunnel: w360 -> [_ w372]
          frame Default {
          }
          frame "Stopped" {
            n132 = call <vilib>:"Destroy.vi"("error in (no error)"=w373, "SMO"=w372) -> ("error out"=w374:errorcluster)  [unwired: 9 in]
          }
        }
        n133 = call <vilib>:"Add State(s) to Queue__jki_lib_state_machine.vi"("State(s) in (\"\")"=w370) -> ("States Out"=w369:string)  [unwired: 14 in]
      }
      frame "SMO: Create Instrument UI" {
        # "Do not put any code in this frame.\n(It is a separator no-op. You can make a copy of this frame to create a new Macro frame)"
        n134 = Unbundle By Name(w381) -> ("Instrument.Oxford1820 UI"=w379:refnum<class "Instrument UI.Oxford1820.lvclass">, "Instrument.Oxford1820"=w375:refnum<class "Instrument.Oxford1820.lvclass">)
        n135 = call <userlib>:"Create UI.vi"("error in (no error)"=w377, "Instrument in"=w375, "Instrument UI"=w379) -> ("error out"=w376:errorcluster, "Instrument UI out"=w378:refnum<class "Instrument UI.Oxford1820.lvclass">)  [unwired: 7 in]
        n136 = Bundle By Name(cluster=w381, "Instrument.Oxford1820 UI"=w378) -> (w380:T4)
        n137 = call <vilib>:"Add State(s) to Queue__jki_lib_state_machine.vi"("State(s) in (\"\")"=w384) -> ("States Out"=w383:string)  [unwired: 14 in]
      }
      frame "SMO: Start Instrument UI" {
        # "Do not put any code in this frame.\n(It is a separator no-op. You can make a copy of this frame to create a new Macro frame)"
        n138 = Unbundle By Name(w388) -> ("Instrument.Oxford1820 UI"=w387:refnum<class "Instrument UI.Oxford1820.lvclass">)
        n139 = call <vilib>:"Start.vi"("error in (no error)"=w386, "SMO"=w387) -> ("error out"=w385:errorcluster)  [unwired: 8 in, 1 out]
        n140 = call <vilib>:"Add State(s) to Queue__jki_lib_state_machine.vi"("State(s) in (\"\")"=w391) -> ("States Out"=w390:string)  [unwired: 14 in]
      }
      frame "SMO: Show Instrument UI" {
        # "Do not put any code in this frame.\n(It is a separator no-op. You can make a copy of this frame to create a new Macro frame)"
        n141 = Unbundle By Name(w399) -> ("Instrument.Oxford1820 UI"=w397:refnum<class "Instrument UI.Oxford1820.lvclass">)
        n142 = call <vilib>:"GetState.vi"("error in (no error)"=w395, "SMO"=w397) -> ("error out"=w393:errorcluster, "SMO State"=w392:T1, "SMO out"=w396:refnum<class "Instrument UI.Oxford1820.lvclass">)  [unwired: 7 in]
        n143 = call <vilib>:"Clear Errors.vi"("error in (no error)"=w393) -> ("error out"=w394:errorcluster)  [unwired: 5 in, 1 out]
        n144 = case shown="\"Started\"" w392 {
          tunnel: [w403 w406] -> w398
          tunnel: w396 -> [_ w405]
          tunnel: w394 -> [w403 w404]
          frame Default {
          }
          frame "Started" {
            n145 = call <vilib>:"Show.vi"("error in (no error)"=w404, "SMO.UI"=w405) -> ("error out"=w406:errorcluster)  [unwired: 8 in, 1 out]
          }
        }
        n146 = call <vilib>:"Add State(s) to Queue__jki_lib_state_machine.vi"("State(s) in (\"\")"=w402) -> ("States Out"=w401:string)  [unwired: 14 in]
      }
      frame "SMO: Hide Instrument UI" {
        # "Do not put any code in this frame.\n(It is a separator no-op. You can make a copy of this frame to create a new Macro frame)"
        n147 = Unbundle By Name(w414) -> ("Instrument.Oxford1820 UI"=w412:refnum<class "Instrument UI.Oxford1820.lvclass">)
        n148 = call <vilib>:"GetState.vi"("error in (no error)"=w410, "SMO"=w412) -> ("error out"=w408:errorcluster, "SMO State"=w407:T1, "SMO out"=w411:refnum<class "Instrument UI.Oxford1820.lvclass">)  [unwired: 7 in]
        n149 = call <vilib>:"Clear Errors.vi"("error in (no error)"=w408) -> ("error out"=w409:errorcluster)  [unwired: 5 in, 1 out]
        n150 = case shown="\"Started\"" w407 {
          tunnel: [w418 w421] -> w413
          tunnel: w411 -> [_ w420]
          tunnel: w409 -> [w418 w419]
          frame Default {
          }
          frame "Started" {
            n151 = call <vilib>:"Hide.vi"("error in (no error)"=w419, "SMO.UI"=w420) -> ("error out"=w421:errorcluster)  [unwired: 8 in, 1 out]
          }
        }
        n152 = call <vilib>:"Add State(s) to Queue__jki_lib_state_machine.vi"("State(s) in (\"\")"=w417) -> ("States Out"=w416:string)  [unwired: 14 in]
      }
      frame "SMO: Stop Instrument UI" {
        # "Do not put any code in this frame.\n(It is a separator no-op. You can make a copy of this frame to create a new Macro frame)"
        n153 = Unbundle By Name(w428) -> ("Instrument.Oxford1820 UI"=w423:refnum<class "Instrument UI.Oxford1820.lvclass">)
        n154 = call <vilib>:"GetState.vi"("error in (no error)"=w427, "SMO"=w423) -> ("error out"=w426:errorcluster, "SMO State"=w424:T1, "SMO out"=w422:refnum<class "Instrument UI.Oxford1820.lvclass">)  [unwired: 7 in]
        n155 = call <vilib>:"Clear Errors.vi"("error in (no error)"=w426) -> ("error out"=w425:errorcluster)  [unwired: 5 in, 1 out]
        n156 = case shown="\"Created\", \"Started\"" w424 {
          tunnel: [w433 w436] -> w429
          tunnel: w422 -> [_ w435]
          tunnel: w425 -> [w433 w434]
          frame Default {
          }
          frame "Created", "Started" {
            n157 = call <vilib>:"Stop.vi"("error in (no error)"=w434, "SMO"=w435) -> ("error out"=w436:errorcluster)  [unwired: 8 in, 1 out]
          }
        }
        n158 = call <vilib>:"Add State(s) to Queue__jki_lib_state_machine.vi"("State(s) in (\"\")"=w432) -> ("States Out"=w431:string)  [unwired: 14 in]
      }
      frame "SMO: Destroy Instrument UI" {
        # "Do not put any code in this frame.\n(It is a separator no-op. You can make a copy of this frame to create a new Macro frame)"
        n159 = Unbundle By Name(w443) -> ("Instrument.Oxford1820 UI"=w442:refnum<class "Instrument UI.Oxford1820.lvclass">)
        n160 = call <vilib>:"GetState.vi"("error in (no error)"=w440, "SMO"=w442) -> ("error out"=w439:errorcluster, "SMO State"=w437:T1, "SMO out"=w441:refnum<class "Instrument UI.Oxford1820.lvclass">)  [unwired: 7 in]
        n161 = call <vilib>:"Clear Errors.vi"("error in (no error)"=w439) -> ("error out"=w438:errorcluster)  [unwired: 5 in, 1 out]
        n162 = case shown="\"Stopped\"" w437 {
          tunnel: w438 -> [w448 w451]
          tunnel: [w448 w450] -> w444
          tunnel: w441 -> [_ w449]
          frame Default {
          }
          frame "Stopped" {
            n163 = call <vilib>:"Destroy.vi"("error in (no error)"=w451, "SMO"=w449) -> ("error out"=w450:errorcluster)  [unwired: 9 in]
          }
        }
        n164 = call <vilib>:"Add State(s) to Queue__jki_lib_state_machine.vi"("State(s) in (\"\")"=w447) -> ("States Out"=w446:string)  [unwired: 14 in]
      }
      frame "---------- Splash ----------" {
        # "Template Separator\n(You can make a copy of, or modify, this frame)"
        n165 = call <vilib>:"Add State(s) to Queue__jki_lib_state_machine.vi"("State(s) in (\"\")"=w456) -> ("States Out"=w455:string)  [unwired: 14 in]
      }
      frame "Splash: Set Status" {
        # "Your code here.\n(You can make a copy of, or modify, this frame)"
        n166 = property on="Splash Status" class="Str"(error in=w459, "Value"=w460) -> (error out=w458:errorcluster)  [unwired: 1 in, 1 out]
        n167 = call <vilib>:"Add State(s) to Queue__jki_lib_state_machine.vi"("State(s) in (\"\")"=w463) -> ("States Out"=w462:string)  [unwired: 14 in]
      }
      frame "Splash: 2" {
        # "Your code here.\n(You can make a copy of, or modify, this frame)"
        n168 = call <vilib>:"Add State(s) to Queue__jki_lib_state_machine.vi"("State(s) in (\"\")"=w468) -> ("States Out"=w467:string)  [unwired: 14 in]
      }
    }
  }
  "error out" <- w1
